vi "RegisterImage.vi"(8 "error in":errorcluster, 10 "RegisterImageRoutedMessage data":T2, 11 "config":T1) -> (0 "error out":errorcluster, 3 "config":T1)   [LabVIEW 2017, in "IrDataEventCreator.lvlib"]
uses:
  <vilib>/addons/InsightCM/Devices/Shared/Ir/IrDataEventCreator/IrDataEventCreator.lvlib
  <vilib>/addons/InsightCM/Devices/Shared/Ir/IrDataEventCreator/controls/RegisterImageRoutedMessage.ctl
  <vilib>/addons/InsightCM/Devices/Shared/Ir/IrDataEventCreator/controls/Registry_Image.ctl
  <vilib>/addons/InsightCM/MessageBus/Base/controls/KeyValuePair.ctl
  <vilib>/addons/InsightCM/Devices/Shared/Ir/IrDataEventCreator/controls/config.ctl
  <vilib>/addons/InsightCM/Devices/Shared/Ir/IrDataEventCreator/controls/Registry.ctl
  <vilib>/addons/InsightCM/Devices/Shared/Common/DataEventCreator/controls/Registry_Trend.ctl
  <vilib>/addons/InsightCM/Devices/Shared/Common/DataEventCreator/DataEventCreator.lvlib
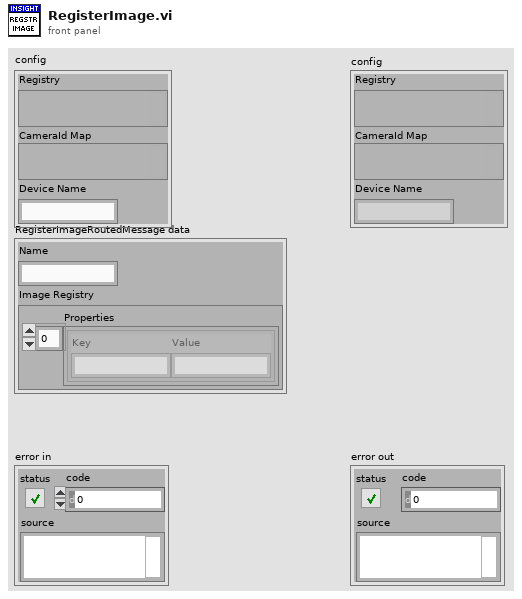
[diagram p1: front panel]
types:
  T1 = typedef "IrDataEventCreator.lvlib/config.ctl" = cluster{"Registry":variant, "CameraId Map":variant, "Device Name":string}
  T2 = typedef "IrDataEventCreator.lvlib/RegisterImageRoutedMessage.ctl" = cluster{"Name":string, "Image Registry":T3}
  T3 = typedef "IrDataEventCreator.lvlib/Registry_Image.ctl" = cluster{"Properties":T4[]}
  T4 = typedef "KeyValuePair.ctl" = cluster{"Key":string, "Value":string}
  T5 = typedef "IrDataEventCreator.lvlib/Registry.ctl" = cluster{"Image":T3, "Trend Points":T6[]}
  T6 = typedef "DataEventCreator.lvlib/Registry_Trend.ctl" = cluster{"TrendPointId":string, "DataSetName":string, "HighRate":bool, "Always Send":bool}
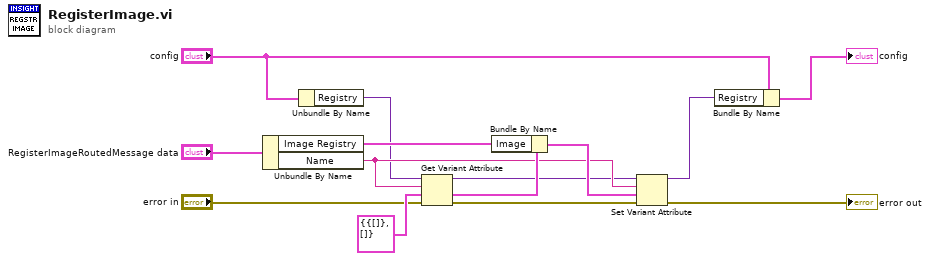
[diagram p0: block diagram]
diagram:
  n1 = Unbundle By Name("RegisterImageRoutedMessage data") -> ("Image Registry"=w9:T3, "Name"=w6:string)
  n2 = Unbundle By Name("config") -> ("Registry"=w4:variant)
  n3 = Get Variant Attribute(Variant=w4, name=w6, default value (empty Variant)=T5 {"Image"={"Properties"=[]}, "Trend Points"=[]} ("Registry"), error in="error in") -> (duplicate Variant=w5:variant, value=w10:T5, error out=w8:errorcluster)  [unwired: 1 out]
  n4 = Bundle By Name(cluster=w10, "Image"=w9) -> (w7:T5)
  n5 = Set Variant Attribute(Variant=w5, name=w6, value=w7, error in=w8) -> (Variant out=w3:variant, error out=→"error out":errorcluster)  [unwired: 1 out]
  n6 = Bundle By Name(cluster="config", "Registry"=w3) -> (→"config":T1)
